vi "create logfile path.vi"(11 "PackedLibrary in":refnum<class "Builder.lvclass">) -> (3 "logfile path":path)   [LabVIEW 2024, in "Builder.lvclass"]
uses:
  packed_library/PackedLibrary.lvclass/PackedLibrary.ctl
  Builder.lvclass
  Builder.lvclass/Builder.ctl
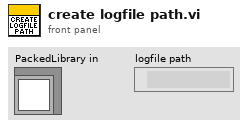
[diagram p1: front panel]
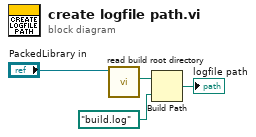
[diagram p0: block diagram]
diagram:
  n1 = call "read build root directory.vi"("Builder in"="PackedLibrary in") -> ("build root directory"=w4:path)  [unwired: 10 in]
  n2 = Build Path(base path=w4, name or relative path=path "build.log") -> (appended path=→"logfile path":path)
